vi "Change DUT Channel.vi"(0 "Data Cluster In":T1={"Message"="", "Homed?"=FALSE, "NextState"=enum."Timeout", "G.Load"=0.0, "G.Position"=0.0, "Load#"=0, "[G.Loads]"=[], "[TotalLoads]"=[], "[Errors]"=[], "ZeroWait"=0, "Results"=[], "DwellWait"=FALSE, "Test Result"=FALSE, "[CondyleLoads]"=[], "[Max]"=[], "[Min]"=[], "Valid String?"=FALSE, "ScanTime"=timestamp(0 s since 1904-01-01), "ScannedString"="", "LabelDevID"=0, "MfgDate"=timestamp(0 s since 1904-01-01), "[EEPROM Cmds]"=[], "[CalData]"=[], "[A/Ds]"=[], "[A/Dmax]"=[], "[A/Dmin]"=[], "BattMax"=0.0, "BattMin"=0.0, "DwellTime"=2000, "PendingDeviceType"="", "Zero G.load"=0.0, "GAINC Value"="", "Programming Step"=enum."Load EEPROM", "Front Panel Program?"=FALSE, "Final Program?"=FALSE, "PCB Score"=100, "AssyScore"=100, "Pass/Fail #"="", "Result String"="", "Programming Mode"=enum."Initial Program", "Angle Test Step"=enum."Initialize", "Accel Values"=[], "Shutdown Counter"=0, "V1"=0, "V2"=0, "V3"=0, "V4"=0, "EEPROM Data"=[], "Counter"=0, "Page#"=0, "Timer"=timestamp(0 s since 1904-01-01), "Use Mark10?"=FALSE, "Eng-Result#"=0, "DUT Serial #"=0, "Scroll Message?"=FALSE, "Clear Message"=FALSE, "Batt Test Step "=enum."Initialize", "RXTX Window Found?"=FALSE, "Shutdown First Call?"=FALSE, "A2 Delay (msec)"=500, "Support Script"={"Script #"="", "Script Revision"="", "[OEMs]"=[], "[[DeviceTypes]]"=[], "[[DeviceTypesVals]]"=[], "[[List of Errors]]"=[], "Default GAINC"="", "[[ASICtrims]]"=[], "ID For Echo"="", "Condyle A CalFactor"=100, "Condyle B CalFactor"=100, "[OEMs Prefix]"=[], "Packet ID 18"="", "[[Force Table Load Test]]"=[], "[[Force Table AccurTest]]"=[]}, "Serial Table"={"Serial File Path"=path "", "[[Serial Lookup Table]]"=[], "Serial Device Info"=[], "Valid Serial?"=FALSE}, "Target Information"={"Target Brand"="", "Target DeviceType"="", "Target Serial#"=100, "Target Lot#"=0, "Target DevID"=0, "Target Channel"=5}, "Operator"="", "COM Port"="", "Config Path"=path "", "Tx Array"=[], "DUT Parameters"={"Channel"=0, "DeviceID"=0, "Script Rev"=0, "Month"=0, "Day"=0, "Year"=0, "Lot#"=0, "V1"=0, "V2"=0, "V3"=0, "V4"=0, "MFG"=0, "Cal FactorA"=0, "Cal FactorB"=0, "ASICtrim"=[], "TmpChan"=0, "GAINC"="", "Brand"="", "Device"="", "Serial #"=0, "Batt310"=0, "Batt 280"=0}, "FTS Main?"=FALSE, "Loading"={"[Forces]"=[], "[Dwell]"=[], "Loading Step"=enum."Initialize Test"}, "Software Version"="", "Correction Factor"="", "Second Load Test"=FALSE, "Acc Loads"=[], "Mark10 Config"={"H2S%"=[80.0, 85.0, 90.0, 95.0, 100.0], "H2S Speed"=[12.0, 8.0, 6.0, 4.0, 2.0], "H to S"=2.0, "Home Speed"=1.0, "LoadWin"=0.0, "Load Speed"=0.0, "PID"={"Kp"=0.04, "Kd"=0.005001, "Ki"=2.9999999999999923e-05}}, "Channels"={"Transceiver Ch"=5, "Operating Ch"=5, "Start Ch"=2}, "Channel EEPROM"=[], "Load Notes"=[], "Engr Log?"=FALSE} {"Mark10 Config"."PID"."Ki" min=0.0 max=200.0 format="%.6f"; "Mark10 Config"."PID"."Kd" min=0.0 max=200.0 format="%.6f"; "Mark10 Config"."PID"."Kp" min=0.0 max=200.0 format="%.6f"; "DUT Parameters"."ASICtrim" format="%02x"}, 11 "error in (no error)":errorcluster) -> (4 "Data Cluster Out":T1={"Message"="", "Homed?"=FALSE, "NextState"=enum."Timeout", "G.Load"=0.0, "G.Position"=0.0, "Load#"=0, "[G.Loads]"=[], "[TotalLoads]"=[], "[Errors]"=[], "ZeroWait"=0, "Results"=[], "DwellWait"=FALSE, "Test Result"=FALSE, "[CondyleLoads]"=[], "[Max]"=[], "[Min]"=[], "Valid String?"=FALSE, "ScanTime"=timestamp(0 s since 1904-01-01), "ScannedString"="", "LabelDevID"=0, "MfgDate"=timestamp(0 s since 1904-01-01), "[EEPROM Cmds]"=[], "[CalData]"=[], "[A/Ds]"=[], "[A/Dmax]"=[], "[A/Dmin]"=[], "BattMax"=0.0, "BattMin"=0.0, "DwellTime"=2000, "PendingDeviceType"="", "Zero G.load"=0.0, "GAINC Value"="", "Programming Step"=enum."Load EEPROM", "Front Panel Program?"=FALSE, "Final Program?"=FALSE, "PCB Score"=100, "AssyScore"=100, "Pass/Fail #"="", "Result String"="", "Programming Mode"=enum."Initial Program", "Angle Test Step"=enum."Initialize", "Accel Values"=[], "Shutdown Counter"=0, "V1"=0, "V2"=0, "V3"=0, "V4"=0, "EEPROM Data"=[], "Counter"=0, "Page#"=0, "Timer"=timestamp(0 s since 1904-01-01), "Use Mark10?"=FALSE, "Eng-Result#"=0, "DUT Serial #"=0, "Scroll Message?"=FALSE, "Clear Message"=FALSE, "Batt Test Step "=enum."Initialize", "RXTX Window Found?"=FALSE, "Shutdown First Call?"=FALSE, "A2 Delay (msec)"=500, "Support Script"={"Script #"="", "Script Revision"="", "[OEMs]"=[], "[[DeviceTypes]]"=[], "[[DeviceTypesVals]]"=[], "[[List of Errors]]"=[], "Default GAINC"="", "[[ASICtrims]]"=[], "ID For Echo"="", "Condyle A CalFactor"=100, "Condyle B CalFactor"=100, "[OEMs Prefix]"=[], "Packet ID 18"="", "[[Force Table Load Test]]"=[], "[[Force Table AccurTest]]"=[]}, "Serial Table"={"Serial File Path"=path "", "[[Serial Lookup Table]]"=[], "Serial Device Info"=[], "Valid Serial?"=FALSE}, "Target Information"={"Target Brand"="", "Target DeviceType"="", "Target Serial#"=100, "Target Lot#"=0, "Target DevID"=0, "Target Channel"=5}, "Operator"="", "COM Port"="", "Config Path"=path "", "Tx Array"=[], "DUT Parameters"={"Channel"=0, "DeviceID"=0, "Script Rev"=0, "Month"=0, "Day"=0, "Year"=0, "Lot#"=0, "V1"=0, "V2"=0, "V3"=0, "V4"=0, "MFG"=0, "Cal FactorA"=0, "Cal FactorB"=0, "ASICtrim"=[], "TmpChan"=0, "GAINC"="", "Brand"="", "Device"="", "Serial #"=0, "Batt310"=0, "Batt 280"=0}, "FTS Main?"=FALSE, "Loading"={"[Forces]"=[], "[Dwell]"=[], "Loading Step"=enum."Initialize Test"}, "Software Version"="", "Correction Factor"="", "Second Load Test"=FALSE, "Acc Loads"=[], "Mark10 Config"={"H2S%"=[80.0, 85.0, 90.0, 95.0, 100.0], "H2S Speed"=[12.0, 8.0, 6.0, 4.0, 2.0], "H to S"=2.0, "Home Speed"=1.0, "LoadWin"=0.0, "Load Speed"=0.0, "PID"={"Kp"=0.04, "Kd"=0.005001, "Ki"=2.9999999999999923e-05}}, "Channels"={"Transceiver Ch"=5, "Operating Ch"=5, "Start Ch"=2}, "Channel EEPROM"=[], "Load Notes"=[], "Engr Log?"=FALSE} {"Mark10 Config"."PID"."Ki" min=0.0 max=200.0 format="%.6f"; "Mark10 Config"."PID"."Kd" min=0.0 max=200.0 format="%.6f"; "Mark10 Config"."PID"."Kp" min=0.0 max=200.0 format="%.6f"; "DUT Parameters"."ASICtrim" format="%02x"}, 15 "error out":errorcluster)   [LabVIEW 2013]
uses:
  Controls/LocalVars.ctl
  Controls/Gen2 FT states.ctl
  Controls/Iniial Device Programming.ctl
  ProgramStageControl.ctl
  Controls/Batt Cap Steps.ctl
  Controls/Support Script.ctl
  Controls/Serial Table.ctl
  Controls/Device Information.ctl
  Controls/InfoPacket.ctl
  Controls/Loading.ctl
  Controls/Load Step.ctl
  Controls/Mark10 Config.ctl
  Controls/PID parameters.ctl
  Controls/Channels.ctl
  Controls/Change DUT Channel.ctl
  RxTx/XceiverStates.ctl
  RxTx/XceiverCmds.ctl
  Controls/Gen2 FT Globals.vi
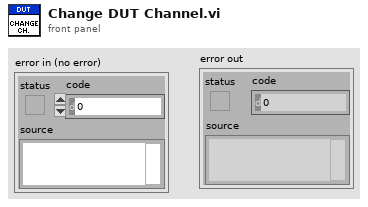
[diagram p1: front panel]
types:
  T1 = typedef "LocalVars.ctl" = cluster{"Message":string, "Homed?":bool, "NextState":T2, "G.Load":dbl, "G.Position":dbl, "Load#":i32, "[G.Loads]":dbl[], "[TotalLoads]":dbl[], "[Errors]":dbl[][], "ZeroWait":u32, "Results":dbl[], "DwellWait":bool, "Test Result":bool, "[CondyleLoads]":dbl[][], "[Max]":dbl[], "[Min]":dbl[], "Valid String?":bool, "ScanTime":timestamp, "ScannedString":string, "LabelDevID":u32, "MfgDate":timestamp, "[EEPROM Cmds]":u8[][], "[CalData]":u8[][], "[A/Ds]":dbl[][], "[A/Dmax]":dbl[], "[A/Dmin]":dbl[], "BattMax":dbl, "BattMin":dbl, "DwellTime":i32, "PendingDeviceType":string, "Zero G.load":dbl, "GAINC Value":string, "Programming Step":T3, "Front Panel Program?":bool, "Final Program?":bool, "PCB Score":i32, "AssyScore":i32, "Pass/Fail #":string, "Result String":string, "Programming Mode":T4, "Angle Test Step":enum16{"Initialize", "Get X", "Get Y", "Get Z", "Next Test"}, "Accel Values":dbl[][], "Shutdown Counter":u32, "V1":i32, "V2":i32, "V3":i32, "V4":i32, "EEPROM Data":i32[][], "Counter":i32, "Page#":i32, "Timer":timestamp, "Use Mark10?":bool, "Eng-Result#":u32, "DUT Serial #":i32, "Scroll Message?":bool, "Clear Message":bool, "Batt Test Step ":T5, "RXTX Window Found?":bool, "Shutdown First Call?":bool, "A2 Delay (msec)":i16, "Support Script":T6, "Serial Table":T7, "Target Information":T8, "Operator":string, "COM Port":string, "Config Path":path, "Tx Array":u8[], "DUT Parameters":T9, "FTS Main?":bool, "Loading":T10, "Software Version":string, "Correction Factor":string, "Second Load Test":bool, "Acc Loads":dbl[][], "Mark10 Config":T12, "Channels":T14, "Channel EEPROM":i32[][], "Load Notes":string[], "Engr Log?":bool}
  T2 = typedef "Gen2 FT states.ctl" = enum16{"---------SETUP-------", "Initialization", "Read Support Data", "Initialize Mark-10", "Initialize Transceiver", "------UTILITIES------", "Change DUT Channel", "Find RxTx Window", "Reset Device", "Scan Channels", "Read Serial Lookup", "Shutdown Device", "ESTOP", "--------USER---------", "Timeout", "-----PROGRAM-----", "Program Device", "------MARK10--------", "Go Home", "MoveUp", "MoveDown", "Goto Load", "Goto Position", "Stop Motor", "---------TESTS--------", "Start Test", "Angle Test", "Load Test", "Load Accuracy Test", "Battery Test", "------RESULTS-------", "End Test", "Display Result", "--------EXIT--------", "Exit"}
  T3 = typedef "Iniial Device Programming.ctl" = enum16{"Load EEPROM", "Send First A1", "Send EEPROM", "Send A1", "Check EEPROM Echo", "Verify transmission", "Programming Successful", "Programming Failed"}
  T4 = typedef "ProgramStageControl.ctl" = enum16{"Initial Program", "GainC", "Scales"}
  T5 = typedef "Batt Cap Steps.ctl" = enum16{"Initialize", "Collect 2.8 Volts", "Collect 3.1 Volts", "Check Results"}
  T6 = typedef "Support Script.ctl" = cluster{"Script #":string, "Script Revision":string, "[OEMs]":string[], "[[DeviceTypes]]":string[][], "[[DeviceTypesVals]]":u16[][], "[[List of Errors]]":string[][], "Default GAINC":string, "[[ASICtrims]]":u8[][], "ID For Echo":string, "Condyle A CalFactor":i32, "Condyle B CalFactor":i32, "[OEMs Prefix]":string[], "Packet ID 18":string, "[[Force Table Load Test]]":dbl[][], "[[Force Table AccurTest]]":dbl[][]}
  T7 = typedef "Serial Table.ctl" = cluster{"Serial File Path":path, "[[Serial Lookup Table]]":string[][], "Serial Device Info":string[], "Valid Serial?":bool}
  T8 = typedef "Device Information.ctl" = cluster{"Target Brand":string, "Target DeviceType":string, "Target Serial#":i32, "Target Lot#":u32, "Target DevID":u32, "Target Channel":u8}
  T9 = typedef "InfoPacket.ctl" = cluster{"Channel":u8, "DeviceID":u32, "Script Rev":u8, "Month":u8, "Day":u8, "Year":u8, "Lot#":u32, "V1":u16, "V2":u16, "V3":u16, "V4":u16, "MFG":u8, "Cal FactorA":u8, "Cal FactorB":u8, "ASICtrim":u8[], "TmpChan":u8, "GAINC":string, "Brand":string, "Device":string, "Serial #":u64, "Batt310":u16, "Batt 280":u16}
  T10 = typedef "Loading.ctl" = cluster{"[Forces]":dbl[], "[Dwell]":dbl[], "Loading Step":T11}
  T11 = typedef "Load Step.ctl" = enum16{"Initialize Test", "Go Home", "Detect Dev Surface", "Wait to zero Device", "Zero Device", "Do Test", "Test Result"}
  T12 = typedef "Mark10 Config.ctl" = cluster{"H2S%":dbl[], "H2S Speed":dbl[], "H to S":dbl, "Home Speed":dbl, "LoadWin":dbl, "Load Speed":dbl, "PID":T13}
  T13 = typedef "PID parameters.ctl" = cluster{"Kp":dbl, "Kd":dbl, "Ki":dbl}
  T14 = typedef "Channels.ctl" = cluster{"Transceiver Ch":u8, "Operating Ch":u8, "Start Ch":u8}
  T15 = typedef "Change DUT Channel.ctl" = enum16{"Initialize", "Send First A1", "Send EEPROM", "Check EEPROM ECHO", "Send A1", "Send A2", "Verify Transmission", "Success", "Failed"}
  T16 = typedef "XceiverStates.ctl" = enum16{"Initialize", "Rx", "Tx", "Raw Mode", "Clear Buffer", "ClearEcho", "Read Buffer", "Close"}
  T17 = typedef "XceiverCmds.ctl" = enum8{"Get Window", "Set Window", "Load&Xmit", "Find Window", "Load CC1101", "Blink LED1", "Blink LED2", "Gen2 Mode", "Request Rev", "Gen2 Mode & Req Rev", "Load Device Settings", "Reset Xceiver", "Set Channel", "Read Channel"}
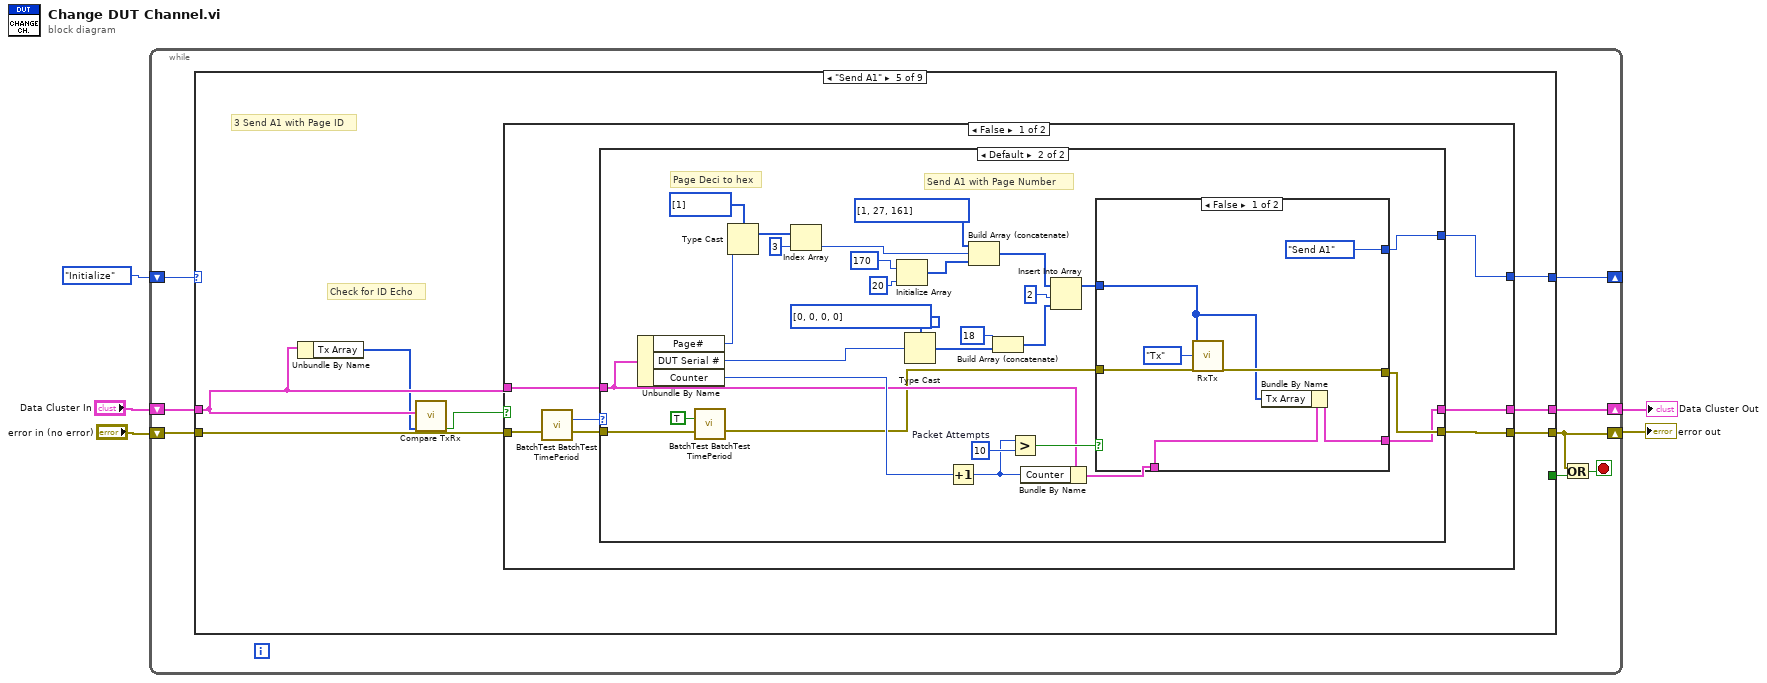
[diagram p0: block diagram]
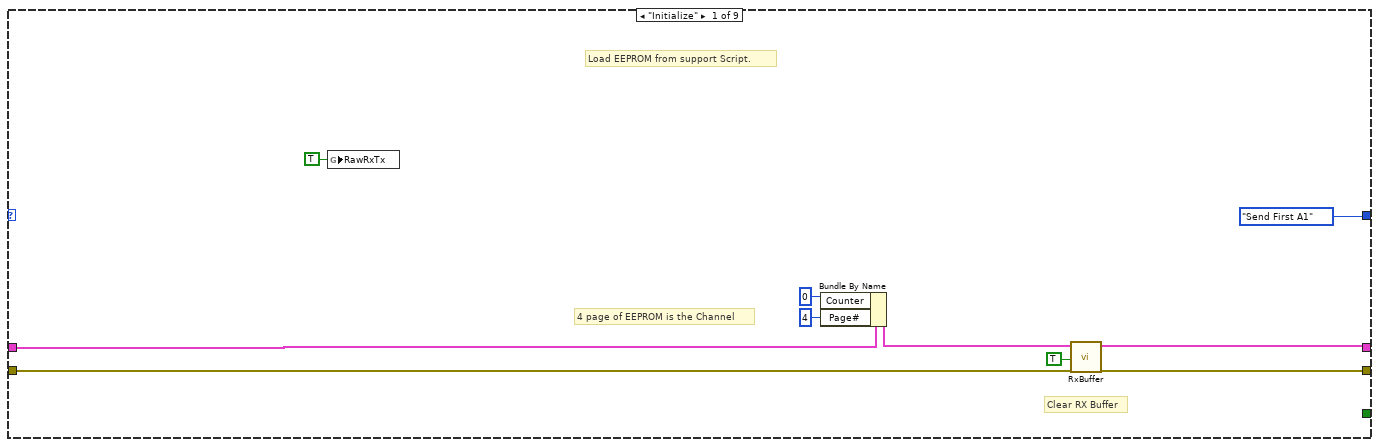
[diagram p2: hidden frame]
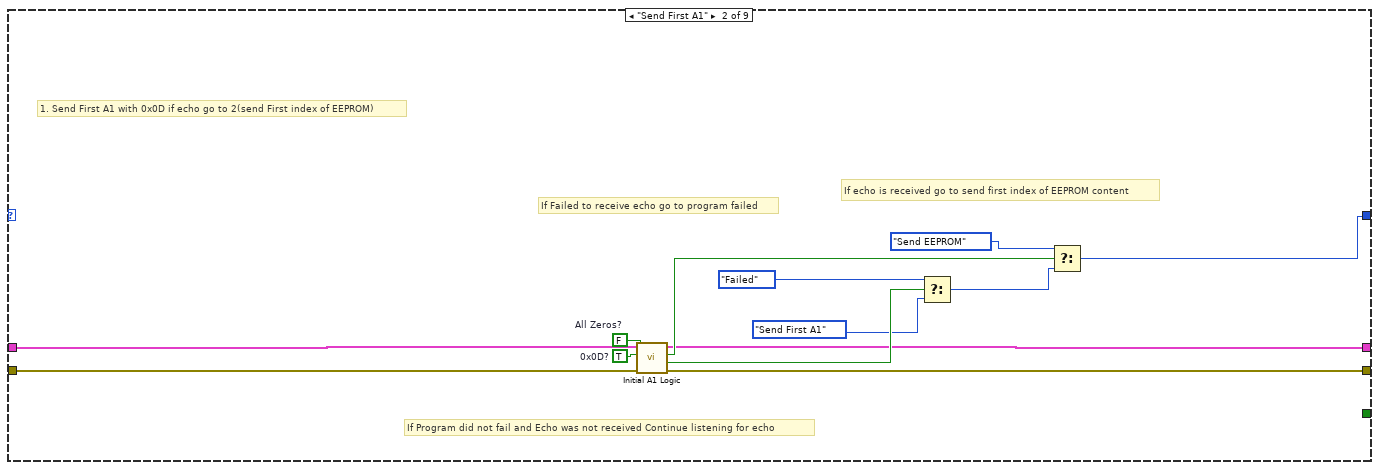
[diagram p3: hidden frame]
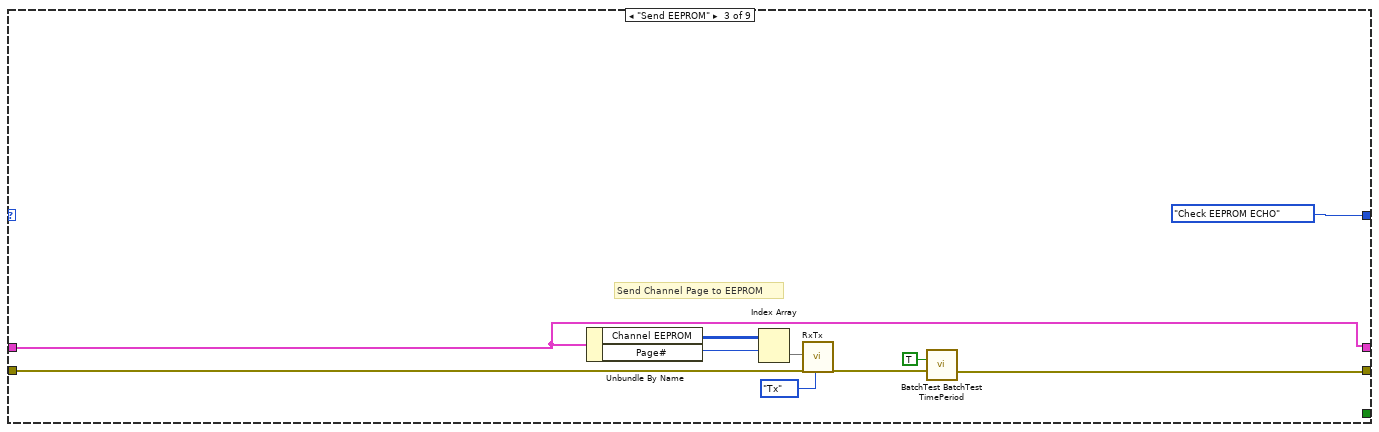
[diagram p4: hidden frame]
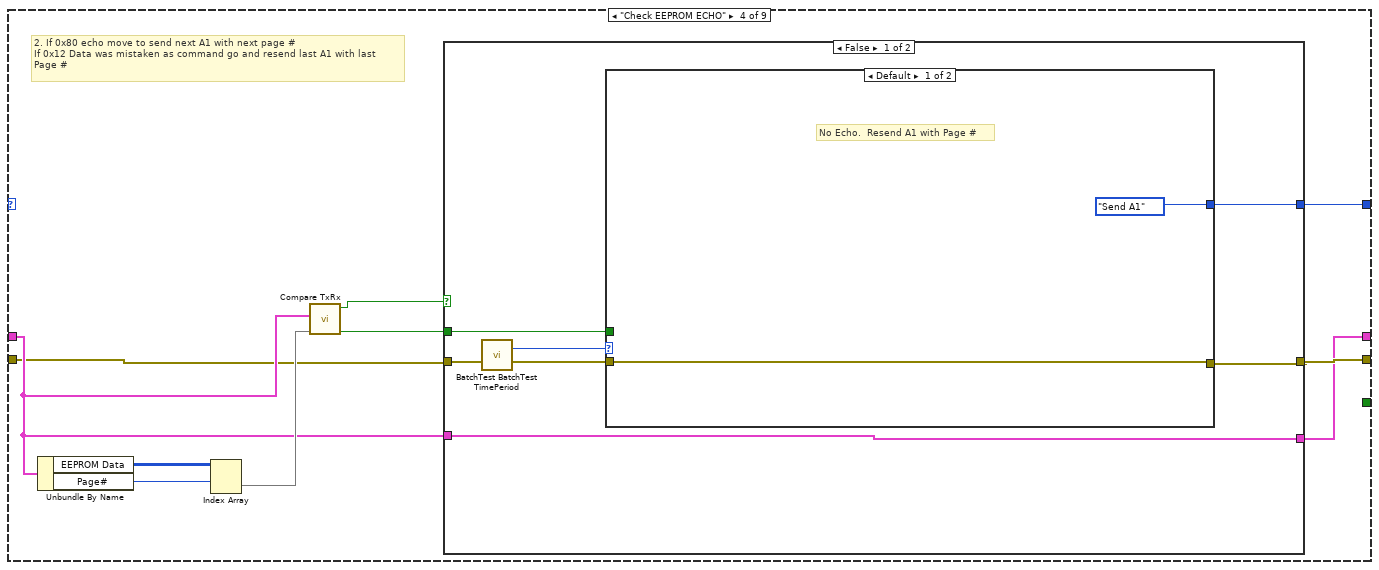
[diagram p5: hidden frame]
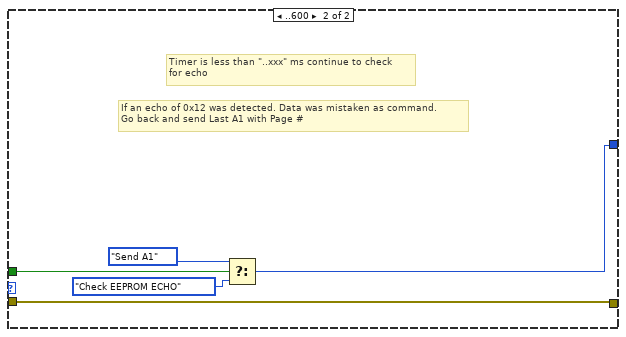
[diagram p6: hidden frame]
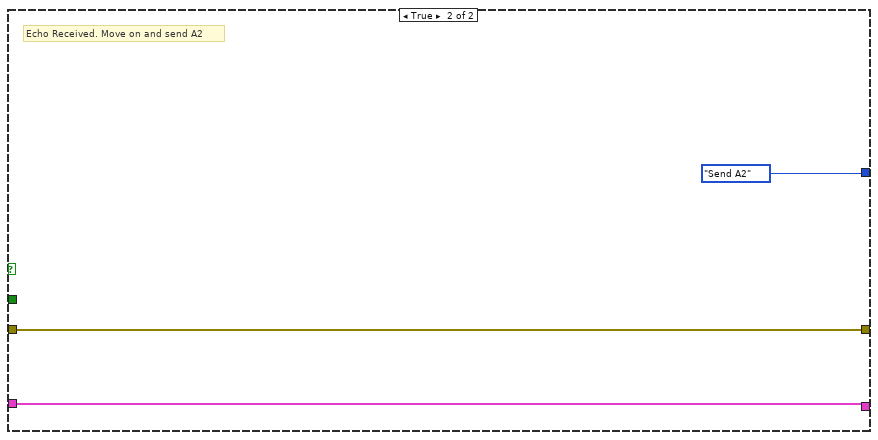
[diagram p7: hidden frame]
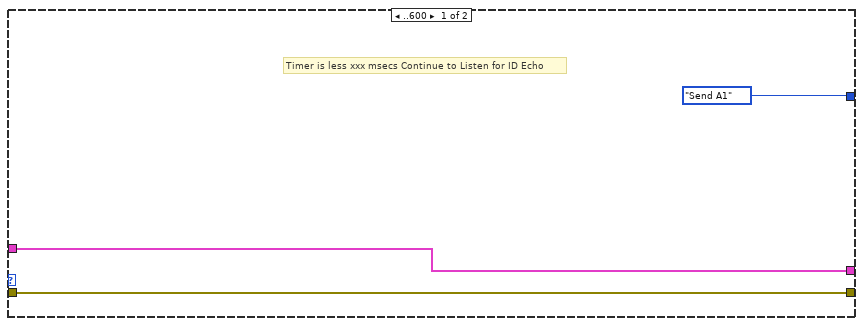
[diagram p8: hidden frame]
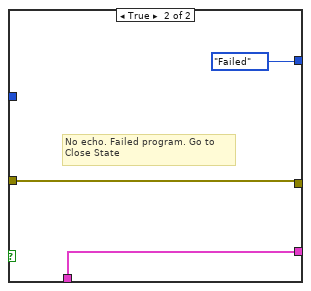
[diagram p9: hidden frame]
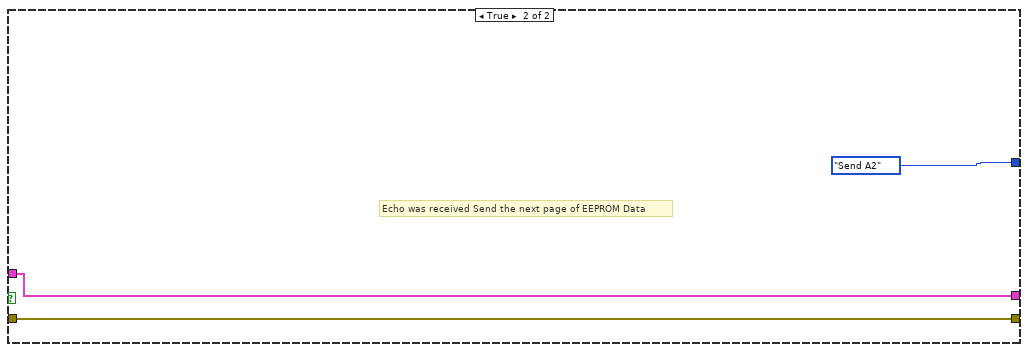
[diagram p10: hidden frame]
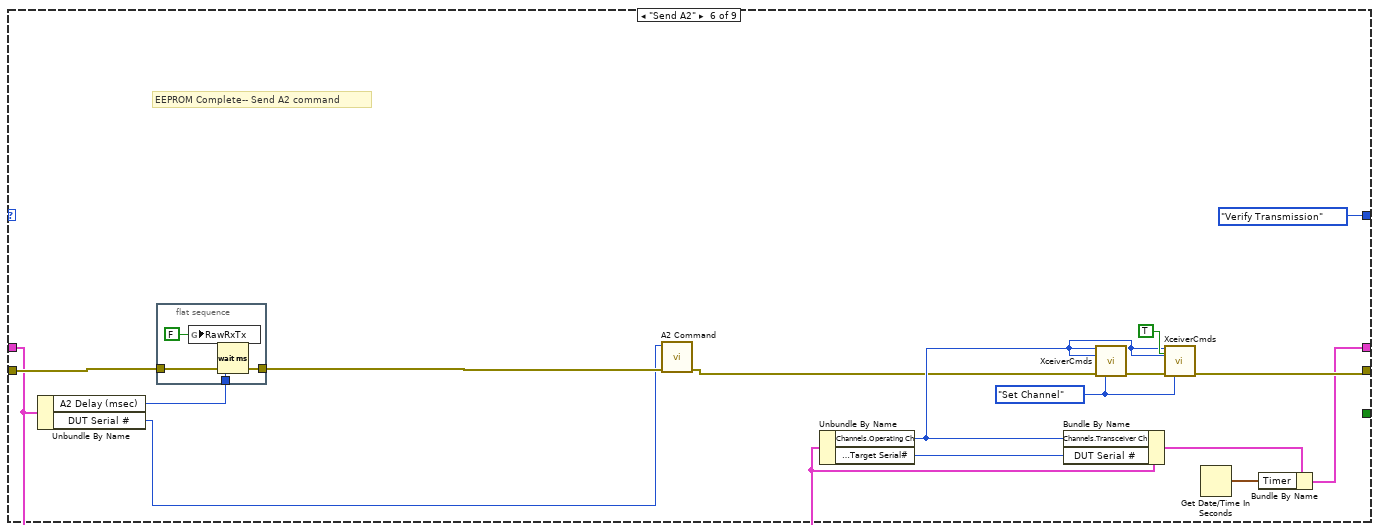
[diagram p11: hidden frame]
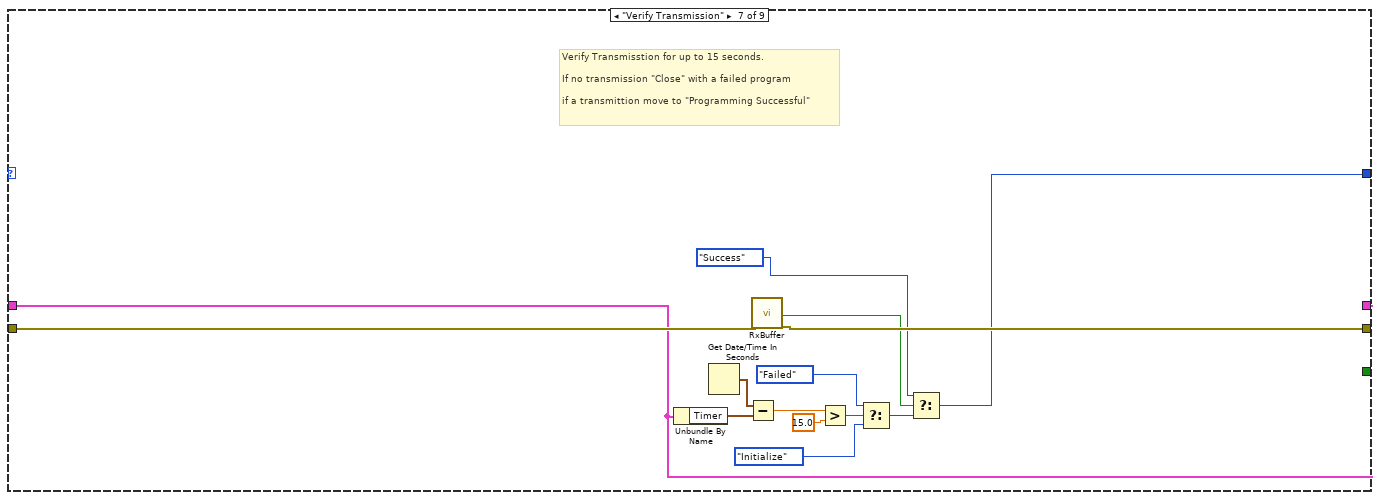
[diagram p12: hidden frame]
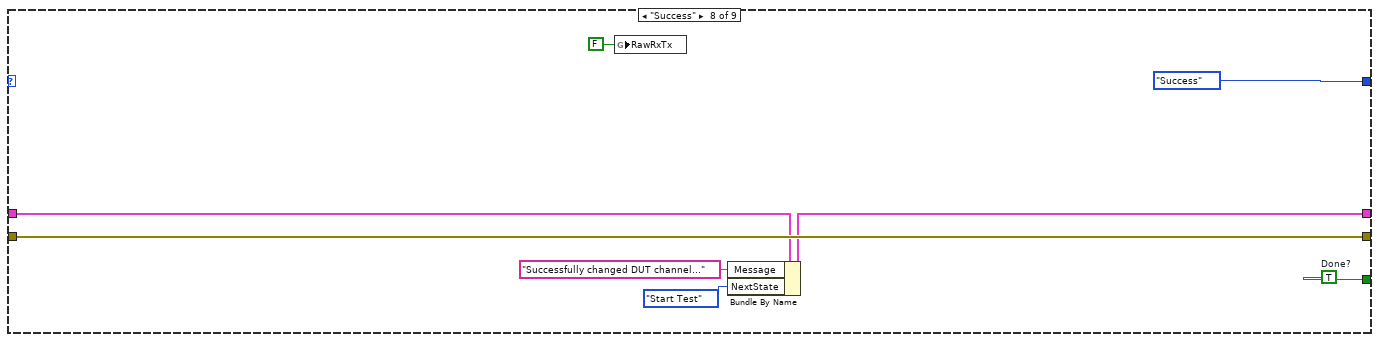
[diagram p13: hidden frame]
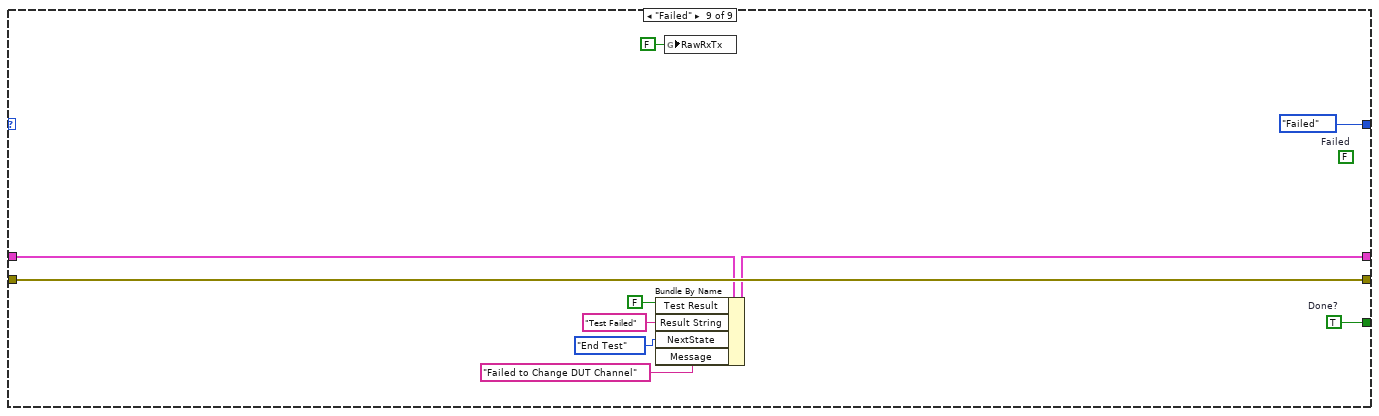
[diagram p14: hidden frame]
diagram:
  n1 = while {
    shift-right: [w7] -> w4
    shift-left: "error in (no error)" -> [w13]
    shift-right: [w12] -> _
    shift-left: Change_DUT_Channel."Initialize" ("State") -> [w9]
    shift-right: [w11] -> w2
    shift-left: "Data Cluster In" -> [w10]
    stop <- w8 stop-if-true
    n2 = case shown="\"Send A1\"" w9 {
      tunnel: [w19 w34 w36 w55 w79 w137 w164 w171 w180] -> w7
      tunnel: w13 -> [w17 w35 w42 w46 w73 w147 w163 w171 w180]
      tunnel: [Change_DUT_Channel."Send First A1" ("State") w30 Change_DUT_Channel."Check EEPROM ECHO" ("State") w54 w78 Change_DUT_Channel."Verify Transmission" ("State") w162 Change_DUT_Channel."Success" ("State") Change_DUT_Channel."Failed" ("State")] -> w12
      tunnel: [_ _ _ _ _ _ _ w172 w182] -> w6
      tunnel: [w22 w28 w41 w50 w77 w135 w155 w167 w177] -> w11
      tunnel: w10 -> [w18 w33 w41 w48 w75 w136 w155 w170 w179]
      frame "Initialize" {
        # "4 page of EEPROM is the Channel"
        # "Load EEPROM from support Script."
        # "Clear RX Buffer"
        n3 = global write "Gen2 FT Globals.vi" "RawRxTx"(TRUE ("Initialize?")) -> ()
        n4 = Bundle By Name(cluster=w18, "Counter"=0, "Page#"=4) -> (w22:T1)
        n5 = call "RxBuffer.vi"("Clear?"=TRUE, "error in (no error)"=w17) -> ("error out"=w19:errorcluster)  [unwired: 7 in, 10 out]
      }
      frame "Send First A1" {
        w26 = FALSE  # All Zeros?
        w27 = TRUE  # 0x0D?
        # "If Program did not fail and Echo was not received Continue listening for echo"
        # "If Failed to receive echo go to program failed"
        # "If echo is received go to send first index of EEPROM content"
        # "1. Send First A1 with 0x0D if echo go to 2(send First index of EEPROM)"
        n6 = call "Initial A1 Logic.vi"("error in (no error)"=w35, "All Zeros?"=w26, "0x0D?"=w27, "Data In"=w33) -> ("error out"=w34:errorcluster, "Failed?"=w32:bool, "Echo?"=w29:bool, "Data Out"=w28:T1)  [unwired: 4 in]
        n7 = Select(t=Change_DUT_Channel."Failed" ("State"), s=w32, f=Change_DUT_Channel."Send First A1" ("State")) -> (s? t:f=w31:T15)
        n8 = Select(t=Change_DUT_Channel."Send EEPROM" ("State"), s=w29, f=w31) -> (s? t:f=w30:T15)
      }
      frame "Send EEPROM" {
        # "Send Channel Page to EEPROM"
        n9 = Unbundle By Name(w41) -> ("Channel EEPROM"=w45:i32[][], "Page#"=w40:i32)
        n10 = Index Array(array=w45, index (row)=w40) -> (element=w43:i32[])  [unwired: 1 in]
        n11 = call "RxTx.vi"("[TxData]"=w43, "error in (no error)"=w42, "Action"=XceiverStates."Tx") -> ("error out"=w38:errorcluster)  [unwired: 8 in, 8 out]
        n12 = call "BatchTest BatchTest TimePeriod.vi"("Initialize?"=TRUE, "error in (no error)"=w38) -> ("error out"=w36:errorcluster)  [unwired: 12 in, 1 out]
      }
      frame "Check EEPROM ECHO" {
        # "2. If 0x80 echo move to send next A1 with next page # \nIf 0x12 Data was mistaken as command go and resend last A1 with last\nPage #"
        n13 = Unbundle By Name(w48) -> ("EEPROM Data"=w53:i32[][], "Page#"=w47:i32)
        n14 = Index Array(array=w53, index (row)=w47) -> (element=w51:i32[])  [unwired: 1 in]
        n15 = call "Compare TxRx.vi"("RawTx"=w51, "Data Cluster In"=w48) -> ("0x12 + Content?"=w49:bool, "0x80 + Content?"=w52:bool)  [unwired: 7 in, 1 out]
        n16 = case shown="False" w52 {
          tunnel: [w60 w72] -> w55
          tunnel: w46 -> [w62 w72]
          tunnel: [w61 Change_DUT_Channel."Send A2" ("State")] -> w54
          tunnel: w48 -> [w57 w71]
          tunnel: [w57 w71] -> w50
          tunnel: w49 -> [w56 _]
          frame False {
            n17 = call "BatchTest BatchTest TimePeriod.vi"("error in (no error)"=w62) -> ("Time(mS)"=w58:u32, "error out"=w59:errorcluster)  [unwired: 13 in]
            n18 = case shown="Default" w58 {
              tunnel: [Change_DUT_Channel."Send A1" ("State") w67] -> w61
              tunnel: [w64 w69] -> w60
              tunnel: w59 -> [w64 w69]
              tunnel: w56 -> [_ w68]
              frame Default {
                # "No Echo.  Resend A1 with Page #"
              }
              frame ..600 {
                # "If an echo of 0x12 was detected. Data was mistaken as command. \nGo back and send Last A1 with Page #"
                # "Timer is less than \"..xxx\" ms continue to check \nfor echo"
                n19 = Select(t=Change_DUT_Channel."Send A1" ("State"), s=w68, f=Change_DUT_Channel."Check EEPROM ECHO" ("State")) -> (s? t:f=w67:T15)
              }
            }
          }
          frame True {
            # "Echo Received. Move on and send A2"
          }
        }
      }
      frame "Send A1" {
        # "3 Send A1 with Page ID"
        # "Check for ID Echo"
        n20 = Unbundle By Name(w75) -> ("Tx Array"=w74:u8[])
        n21 = call "Compare TxRx.vi"("RawTx"=w74, "Data Cluster In"=w75) -> ("0x12 + Content?"=w76:bool)  [unwired: 7 in, 2 out]
        n22 = case shown="False" w76 {
          tunnel: [w85 w131] -> w79
          tunnel: w73 -> [w86 w131]
          tunnel: [w84 Change_DUT_Channel."Send A2" ("State")] -> w78
          tunnel: w75 -> [w82 w129]
          tunnel: [w81 w129] -> w77
          frame False {
            n23 = call "BatchTest BatchTest TimePeriod.vi"("error in (no error)"=w86) -> ("Time(mS)"=w80:u32, "error out"=w83:errorcluster)  [unwired: 13 in]
            n24 = case shown="Default" w80 {
              tunnel: w83 -> [w89 w117]
              tunnel: [w89 w102] -> w85
              tunnel: [Change_DUT_Channel."Send A1" ("State") w101] -> w84
              tunnel: w82 -> [w88 w112]
              tunnel: [w88 w90] -> w81
              frame ..600 {
                # "Timer is less xxx msecs Continue to Listen for ID Echo"
              }
              frame Default {
                w116 = 10  # Packet Attempts
                # "Page Deci to hex"
                # "Send A1 with Page Number"
                n25 = Unbundle By Name(w112) -> ("Page#"=w93:i32, "DUT Serial #"=w100:i32, "Counter"=w115:i32)
                n26 = call "BatchTest BatchTest TimePeriod.vi"("Initialize?"=TRUE, "error in (no error)"=w117) -> ("error out"=w103:errorcluster)  [unwired: 12 in, 1 out]
                n27 = Type Cast(type=u8[] [1], x=w93) -> (*(type *) &x=w95:u8[])
                n28 = Index Array(array=w95, index=3) -> (element=w92:u8)
                n29 = Initialize Array(u8 170, 20 ("dimension size")) -> (w108:u8[])
                n30 = Type Cast(type=u8[] [0, 0, 0, 0] ("initialized array"), x=w100) -> (*(type *) &x=w109:u8[])
                n31 = Increment(x=w115) -> (x+1=w113:i32)
                n32 = Build Array (concatenate)(u8[] [1, 27, 161], w92, w108) -> (w107:u8[])
                n33 = Build Array (concatenate)(u8 18, w109) -> (w105:u8[])
                n34 = Greater?(x=w113, y=w116) -> (0:w114:bool)
                n35 = Bundle By Name(cluster=w112, "Counter"=w113) -> (w91:T1)
                n36 = Insert Into Array(array=w107, index=2, new element=w105) -> (w104:u8[])
                n37 = case shown="False" w114 {
                  tunnel: [Change_DUT_Channel."Send A1" ("State") Change_DUT_Channel."Failed" ("State")] -> w101
                  tunnel: w103 -> [w124 w128]
                  tunnel: [w123 w128] -> w102
                  tunnel: w104 -> [w120 _]
                  tunnel: w91 -> [w122 w127]
                  tunnel: [w121 w127] -> w90
                  frame False {
                    n38 = call "RxTx.vi"("[TxData]"=w120, "error in (no error)"=w124, "Action"=XceiverStates."Tx") -> ("error out"=w123:errorcluster)  [unwired: 8 in, 8 out]
                    n39 = Bundle By Name(cluster=w122, "Tx Array"=w120) -> (w121:T1)
                  }
                  frame True {
                    # "No echo. Failed program. Go to \nClose State"
                  }
                }
              }
            }
          }
          frame True {
            # "Echo was received Send the next page of EEPROM Data"
          }
        }
      }
      frame "Send A2" {
        w143 = TRUE ("RF Chip0 Enable")
        w142 = XceiverCmds."Set Channel" ("XceiverCmd")
        # "EEPROM Complete-- Send A2 command"
        n40 = Unbundle By Name(w136) -> ("A2 Delay (msec)"=w146:i16, "DUT Serial #"=w132:i32)
        n41 = flat-sequence {
          tunnel: w147 -> [w149]
          tunnel: [w149] -> w134
          tunnel: w146 -> [w148]
          frame #0 {
            n42 = global write "Gen2 FT Globals.vi" "RawRxTx"(FALSE ("RawRxTx")) -> ()
            n43 = Wait (ms)(milliseconds to wait=w148) -> ()  [unwired: 1 out]
          }
        }
        n44 = call "A2 Command.vi"("error in (no error)"=w134, "DUT Serial #"=w132) -> ("error out"=w133:errorcluster)  [unwired: 9 in]
        n45 = Unbundle By Name(w136) -> ("Channels.Operating Ch"=w138:u8, "Target Information.Target Serial#"=w139:i32)
        n46 = Bundle By Name(cluster=w136, "Channels.Transceiver Ch"=w138, "DUT Serial #"=w139) -> (w140:T1)
        n47 = call "XceiverCmds.vi"("RF Chip0 Channel"=w138, "RF Chip1 Channel"=w138, "error in (no error)"=w133, "XceiverCmd"=w142) -> ("error out"=w141:errorcluster)  [unwired: 9 in, 2 out]
        n48 = call "XceiverCmds.vi"("RF Chip0 Channel"=w138, "RF Chip0 Enable"=w143, "RF Chip1 Enable"=w143, "RF Chip1 Channel"=w138, "error in (no error)"=w141, "XceiverCmd"=w142) -> ("error out"=w137:errorcluster)  [unwired: 7 in, 2 out]
        n49 = Get Date/Time In Seconds() -> (seconds since 1Jan1904=w144:timestamp)
        n50 = Bundle By Name(cluster=w140, "Timer"=w144) -> (w135:T1)
      }
      frame "Verify Transmission" {
        # "Verify Transmisstion for up to 15 seconds. \n\nIf no transmission \"Close\" with a failed program\n\nif a transmittion move to \"Programming Successful\""
        n51 = Unbundle By Name(w155) -> ("Timer"=w156:timestamp)
        n52 = Get Date/Time In Seconds() -> (seconds since 1Jan1904=w160:timestamp)
        n53 = Subtract(x=w160, y=w156) -> (x-y=w158:dbl)
        n54 = call "RxBuffer.vi"("error in (no error)"=w163) -> ("New Data"=w154:bool, "error out"=w164:errorcluster)  [unwired: 8 in, 9 out]
        n55 = Greater?(x=w158, y=15.0) -> (0:w157:bool)
        n56 = Select(t=Change_DUT_Channel."Failed" ("State"), s=w157, f=Change_DUT_Channel."Initialize" ("State")) -> (s? t:f=w161:T15)
        n57 = Select(t=Change_DUT_Channel."Success" ("State"), s=w154, f=w161) -> (s? t:f=w162:T15)
      }
      frame "Success" {
        w172 = TRUE  # Done?
        n58 = global write "Gen2 FT Globals.vi" "RawRxTx"(FALSE ("RawRxTx")) -> ()
        n59 = Bundle By Name(cluster=w170, "Message"="Successfully changed DUT channel...", "NextState"=Gen2_FT_states."Start Test") -> (w167:T1)
      }
      frame "Failed" {
        (unwired) FALSE  # Failed
        w182 = TRUE  # Done?
        n60 = Bundle By Name(cluster=w179, "Test Result"=FALSE, "Result String"="Test Failed", "NextState"=Gen2_FT_states."End Test", "Message"="Failed to Change DUT Channel") -> (w177:T1)
        n61 = global write "Gen2 FT Globals.vi" "RawRxTx"(FALSE ("RawRxTx")) -> ()
      }
    }
    n62 = Or(x=w7, y=w6) -> (x .or. y?=w8:bool)
  }
  "error out" <- w4
  "Data Cluster Out" <- w2
